vi "(SubVI) chnage name.vi"(9 "replace \".csv\" to":string, 10 "Create path?":bool, 11 "Folder path":path) -> (3 "created path":path)   [LabVIEW 2016]
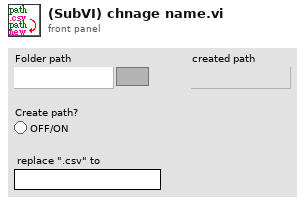
[diagram p1: front panel]
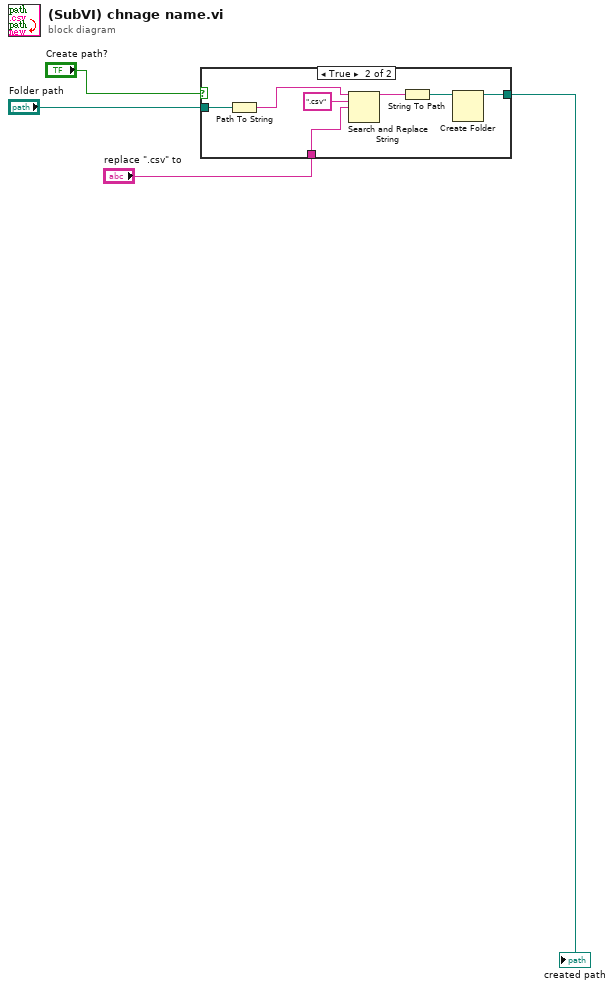
[diagram p0: block diagram]
diagram:
  n1 = case shown="True" "Create path?" {
    tunnel: "Folder path" -> [w5 w12]
    tunnel: [w5 w7] -> w1
    tunnel: "replace \".csv\" to" -> [_ w6]
    frame False {
    }
    frame True {
      n2 = Path To String(path=w12) -> (string=w11:string)
      n3 = Search and Replace String(input string=w11, search string=".csv", replace string=w6) -> (result string=w9:string)  [unwired: 5 in, 3 out]
      n4 = String To Path(string=w9) -> (path=w8:path)
      n5 = Create Folder(path (use dialog)=w8) -> (created path=w7:path)  [unwired: 2 in, 2 out]
    }
  }
  "created path" <- w1
